vi "RSNRPZ Configure Duty Cycle.vi"(0 "VISA session":refnum<visa-resource-name> caption="VISA resource name", 5 "Channel (1)":i32=1, 7 "Duty Cycle State (F: Off)":bool, 9 "Duty Cycle (1.0 %)":dbl=1.0 format="%.2p", 11 "error in (no error)":errorcluster) -> (4 "dup VISA session":refnum<visa-resource-name> caption="VISA resource name", 15 "error out":errorcluster)   [LabVIEW 2010]
doc: "This VI configures all duty cycle parameters.\n\nRemote-control command(s):\nSENS:CORR:DCYC\nSENS:CORR:DCYC:STAT ON | OFF"
uses:
  rsnrpz_32.dll
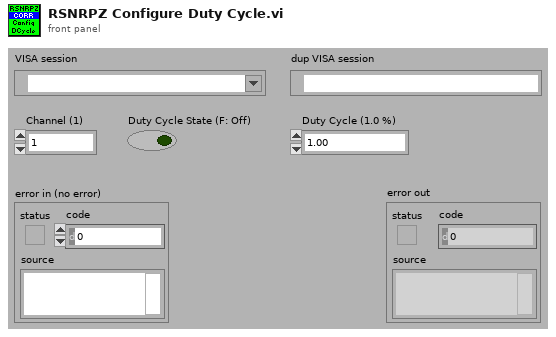
[diagram p1: front panel]
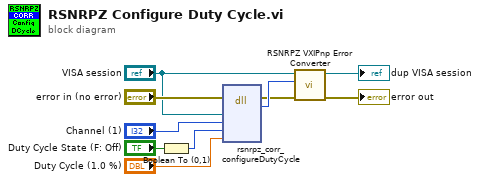
[diagram p0: block diagram]
diagram:
  n1 = Boolean To (0,1)(Boolean="Duty Cycle State (F: Off)") -> (0, 1=w7:i16)
  n2 = dll-call lib="rsnrpz_32.dll" fn="rsnrpz_corr_configureDutyCycle"(error in="error in (no error)", "VISA Session"="VISA session", "Channel"="Channel (1)", "Duty Cycle State"=w7, "Duty Cycle"="Duty Cycle (1.0 %)") -> (error out=w5:errorcluster, "Status"=w9:i32)  [unwired: 6 in, 1 out]
  n3 = call <instrlib>:"RSNRPZ VXIPnp Error Converter.vi"("error in"=w5, "VXIPnp error code"=w9, "VISA session"="VISA session") -> ("error out"=→"error out":errorcluster, "dup VISA session"=→"dup VISA session":refnum<visa-resource-name>)  [unwired: 7 in]
